vi "Format for Tree Control.vi"(8 "Error In":errorcluster, 9 "Class Name":string, 10 "Attr ID":string, 11 "Tree Data":refnum<class "Tree Data.lvclass">) -> (0 "Error Out":errorcluster, 3 "Child Text":string[](array[string]))   [LabVIEW 2017, in "Tree API.lvlib" / "Tree Data.lvclass"]
doc: "This method formats the string data for visualization in Tree Control. For most use cases it can stay default but if you want to have special strings for your own type, override it in child classes of Tree Data."
uses:
  Tree Data.lvclass
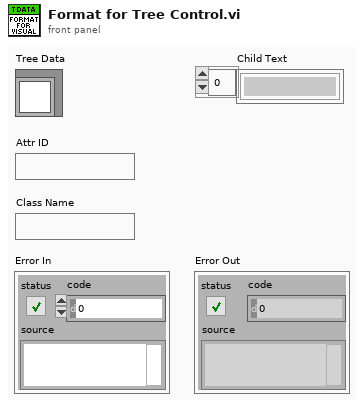
[diagram p1: front panel]
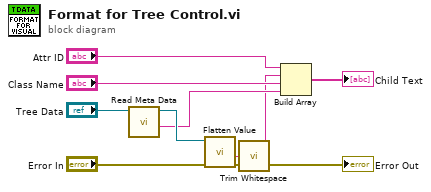
[diagram p0: block diagram]
diagram:
  n1 = call "Read Meta Data.vi"("Tree Data In"="Tree Data") -> ("Meta Data"=w6:string, "Tree Data Out"=w10:refnum<class "Tree Data.lvclass">)  [unwired: 9 in]
  n2 = call-dynamic "Flatten Value.vi"("Error In"="Error In", "Tree Data In"=w10) -> ("Error Out"=→"Error Out":errorcluster, "Value"=w8:string)  [unwired: 7 in, 1 out]
  n3 = call <vilib>:"Trim Whitespace.vi"("string"=w8) -> ("trimmed string"=w1:string)  [unwired: 1 in]
  n4 = Build Array("Attr ID", w1, "Class Name", w6) -> (→"Child Text":string[])
